vi "Test Leak Rate.vi"(7 "Main References":T2, 8 "error in (no error)":errorcluster, 10 "Cart Array":bool[](array[boolean])) -> (0 "error out":errorcluster, 1 "Results":T1[](array[typedef]), 2 "RatePass":bool[](array[boolean]), 3 "VacPass":bool[](array[boolean]))   [LabVIEW 2020]
uses:
  Main Refs.ctl
  Hardware/Tecan/Pump Config.ctl
  Timing Specs.ctl
  Vacuum Specs.ctl
  Cartridges.ctl
  Cartridge Status.ctl
  Commands.ctl
  Lib/Time/Wells.ctl
  Lib/Time/Bottles.ctl
  Process State.ctl
  Vacuum Test.ctl
  Vacuum Output.ctl
  Hardware/Mot Stage Mngr.ctl
  Hardware/Denkovi Mngr.ctl
  Hardware/DAQ Mngr.ctl
panel:
  # "Tecan Pump"
  # "Pressure"
  # "General"
  # "Timing"
  # "Protocol"
  # "Zaber"
  # "NFC Reader 1"
  # "NFC  Reader 2"
  # "NFC Reader 3"
  # "NFC Reader 4"
  # "System"
  # "Cartridge Utitlies"
  # "Wells"
  # "times"
  # "from"
  # "State Machine"
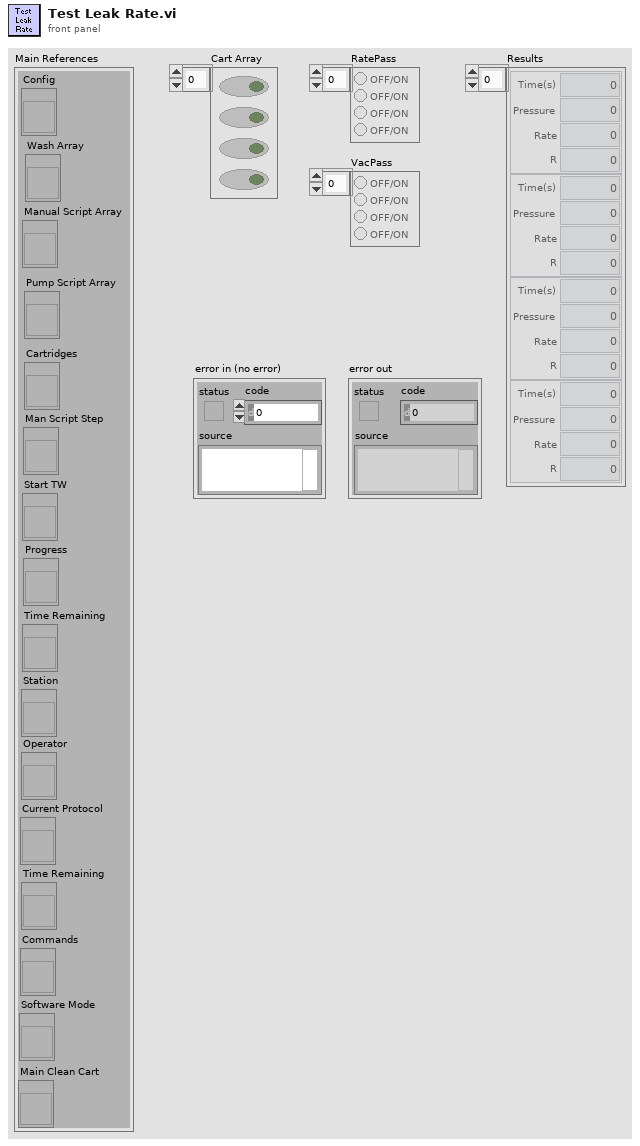
[diagram p1: front panel]
types:
  T1 = typedef "Vacuum Output.ctl" = cluster{"Time(s)":dbl, "Pressure":dbl, "Rate":dbl, "R":dbl}
  T2 = typedef "Main Refs.ctl" = cluster{"Config":refnum<vi>, "Wash Array":refnum<vi>, "Manual Script Array":refnum<vi>, "Pump Script Array":refnum<vi>, "Cartridges":refnum<vi>, "Man Script Step":refnum<vi>, "Start TW":refnum<vi>, "Progress":refnum<vi>, "Time Remaining":refnum<vi>, "Station":refnum<vi>, "Operator":refnum<vi>, "Current Protocol":refnum<vi>, "Time Remaining":refnum<vi>, "Commands":refnum<vi>, "Software Mode":refnum<vi>, "Main Clean Cart":refnum<vi>}
  T3 = typedef "Mot Stage Mngr.ctl" = enum16{"Connect", "Init", "Status", "Send Cmd", "Current Pos", "Set Accel", "Set Max Vel", "Home", "Rel Move", "Abs Move", "Close"}
  T4 = typedef "Denkovi Mngr.ctl" = enum16{"Search", "Init", "Set Peristaltic", "Set Pressure", "Pres ON", "Vent&Close", "Set All Relays", "Set One Relay", "Read Relays", "Close"}
  T5 = typedef "DAQ Mngr.ctl" = enum16{"Init", "Read Pressure", "Analyze Pressure", "Read Cartridges", "Lock Cartridge", "Unlock Cartridge", "Read PS", "Pinch Valve Engage", "Pinch Valve Disengage", "Close"}
  T6 = typedef "Pump Config.ctl" = cluster{"Syringe size":u32, "Syringe address":u32, "# of ports":u32, "Init String":string, "Full Stroke (cnts)":i32, "Model":enum16{"XC", "Centris"}, "TW Position":dbl, "Load Position":dbl, "Bottom Position":dbl, "Station ID":string, "Default Protocol":path, "Dry Time(s)":dbl, "Python Version":string, "NFC SN Array":string[], "Timing":T7, "Pressure Specs":T8}
  T7 = typedef "Timing Specs.ctl" = cluster{"Checking pres and leak":dbl, "Priming input lines":dbl, "Rinsing syringe":dbl, "Filling well X w/ X":dbl, "Drain well X":dbl, "Clearing wells and lines":dbl, "Draining wells":dbl, "Rinsing all wells":dbl, "Testing for leaks/clogs":dbl, "Rinsing wells":dbl}
  T8 = typedef "Vacuum Specs.ctl" = cluster{"Pressure max":dbl, "Pressure min":dbl, "Decay delta":dbl, "Pressure time":dbl, "Conf. R":dbl, "LeakRateMax":dbl}
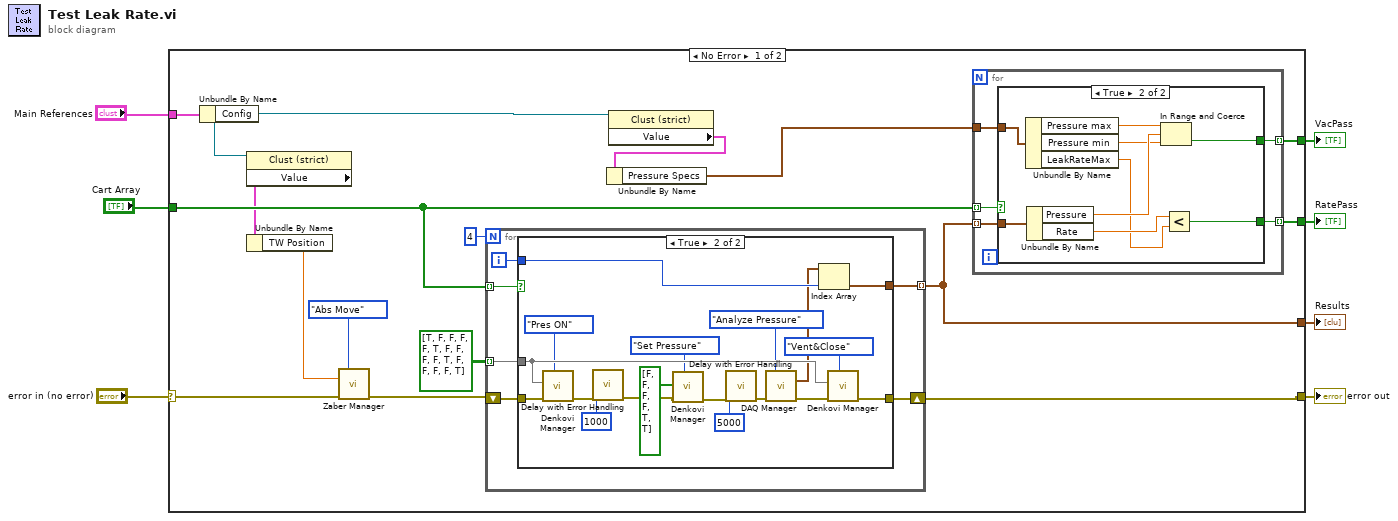
[diagram p0: block diagram]
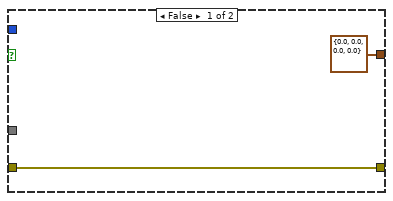
[diagram p2: hidden frame]
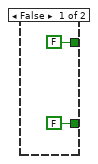
[diagram p3: hidden frame]
diagram:
  n1 = case shown="No Error" "error in (no error)" {
    selector: "error in (no error)" -> [w9 w66]
    tunnel: [w18 w66] -> w6
    tunnel: "Cart Array" -> [w14 _]
    tunnel: "Main References" -> [w23 _]
    tunnel: [w20 _] -> w3
    tunnel: [w19 _] -> w2
    tunnel: [w15 _] -> w1
    frame No Error {
      n2 = Unbundle By Name(w23) -> ("Config"=w12:refnum<vi>)
      n3 = property class="Clust (strict)"(reference=w12) -> ("Value"=w11:T6)  [unwired: 1 in, 2 out]
      n4 = Unbundle By Name(w11) -> ("TW Position"=w10:dbl)
      n5 = call "Zaber Manager.vi"("Action"=Mot_Stage_Mngr."Abs Move", "Value"=w10, "error in (no error)"=w9) -> ("error out"=w8:errorcluster)  [unwired: 6 in, 6 out]
      n6 = for {
        N: 4 -> [_]
        shift-right: [w28] -> w18
        shift-left: w8 -> [w29]
        tunnel: bool[][] [[TRUE, FALSE, FALSE, FALSE], [FALSE, TRUE, FALSE, FALSE], [FALSE, FALSE, TRUE, FALSE], [FALSE, FALSE, FALSE, TRUE]] ("Cart Array") -> [w27] mode=indexing
        tunnel: [w25] -> w15 mode=indexing
        tunnel: w14 -> [w24] mode=indexing
        i -> [w26]
        n7 = case shown="True" w24 {
          tunnel: w29 -> [w30 w49]
          tunnel: [w30 w48] -> w28
          tunnel: w27 -> [_ w47]
          tunnel: w26 -> [_ w46]
          tunnel: [T1 {"Time(s)"=0.0, "Pressure"=0.0, "Rate"=0.0, "R"=0.0} ("Cluster") w45] -> w25
          frame False {
          }
          frame True {
            n8 = call "Denkovi Manager.vi"("Action"=Denkovi_Mngr."Pres ON", "error in (no error)"=w49, "Relays In"=w47) -> ("error out"=w34:errorcluster)  [unwired: 6 in, 2 out]
            n9 = call "Delay with Error Handling.vi"("error in (no error)"=w34, "Delay (ms)"=u32 1000) -> ("error out"=w33:errorcluster)  [unwired: 9 in]
            n10 = call "Denkovi Manager.vi"("Action"=Denkovi_Mngr."Set Pressure", "error in (no error)"=w33, "Relays In"=bool[] [FALSE, FALSE, FALSE, FALSE, TRUE, TRUE]) -> ("error out"=w36:errorcluster)  [unwired: 6 in, 2 out]
            n11 = call "Delay with Error Handling.vi"("error in (no error)"=w36, "Delay (ms)"=u32 5000) -> ("error out"=w42:errorcluster)  [unwired: 9 in]
            n12 = call "DAQ Manager.vi"("DAQ Mngr Action"=DAQ_Mngr."Analyze Pressure", "error in (no error)"=w42) -> ("Data Array"=w32:T1[], "error out"=w40:errorcluster)  [unwired: 7 in, 5 out]
            n13 = Index Array(array=w32, index=w46) -> (element=w45:T1)
            n14 = call "Denkovi Manager.vi"("Action"=Denkovi_Mngr."Vent&Close", "error in (no error)"=w40, "Relays In"=w47) -> ("error out"=w48:errorcluster)  [unwired: 6 in, 2 out]
          }
        }
      }
      n15 = property class="Clust (strict)"(reference=w12) -> ("Value"=w22:T6)  [unwired: 1 in, 2 out]
      n16 = Unbundle By Name(w22) -> ("Pressure Specs"=w21:T8)
      n17 = for {
        tunnel: w15 -> [w53] mode=indexing
        tunnel: w14 -> [w54] mode=indexing
        tunnel: w21 -> [w52]
        tunnel: [w51] -> w20 mode=indexing
        tunnel: [w50] -> w19 mode=indexing
        n18 = case shown="True" w54 {
          tunnel: w53 -> [_ w65]
          tunnel: w52 -> [_ w64]
          tunnel: [FALSE w58] -> w51
          tunnel: [FALSE w57] -> w50
          frame False {
          }
          frame True {
            n19 = Unbundle By Name(w64) -> ("Pressure max"=w60:dbl, "Pressure min"=w59:dbl, "LeakRateMax"=w61:dbl)
            n20 = Unbundle By Name(w65) -> ("Pressure"=w63:dbl, "Rate"=w62:dbl)
            n21 = In Range and Coerce(upper limit=w60, x=w63, lower limit=w59) -> (In Range?=w58:bool)  [unwired: 1 out]
            n22 = Less?(x=w62, y=w61) -> (x < y?=w57:bool)
          }
        }
      }
    }
    frame Error {
    }
  }
  "error out" <- w6
  "VacPass" <- w3
  "RatePass" <- w2
  "Results" <- w1
